vi "Filter_test.vi"(7 "Headers":string[](array[string])=["Packet Number", "Timestamp", "Source", "Destination", "Protocol", "Length", "Data"], 10 "Filter String":string="Protocol == UDP AND Length > 0.7 OR Source == 192.168.1.1", 11 "Prefiltered Data":string[][](array[string])=array1500x7[10500 elements]) -> (0 "Error Out":errorcluster, 3 "Filtered Array":string[][](array[string]))   [LabVIEW 2025, in "Table_Filtering.lvlib"]
uses:
  Table_Filtering.lvlib
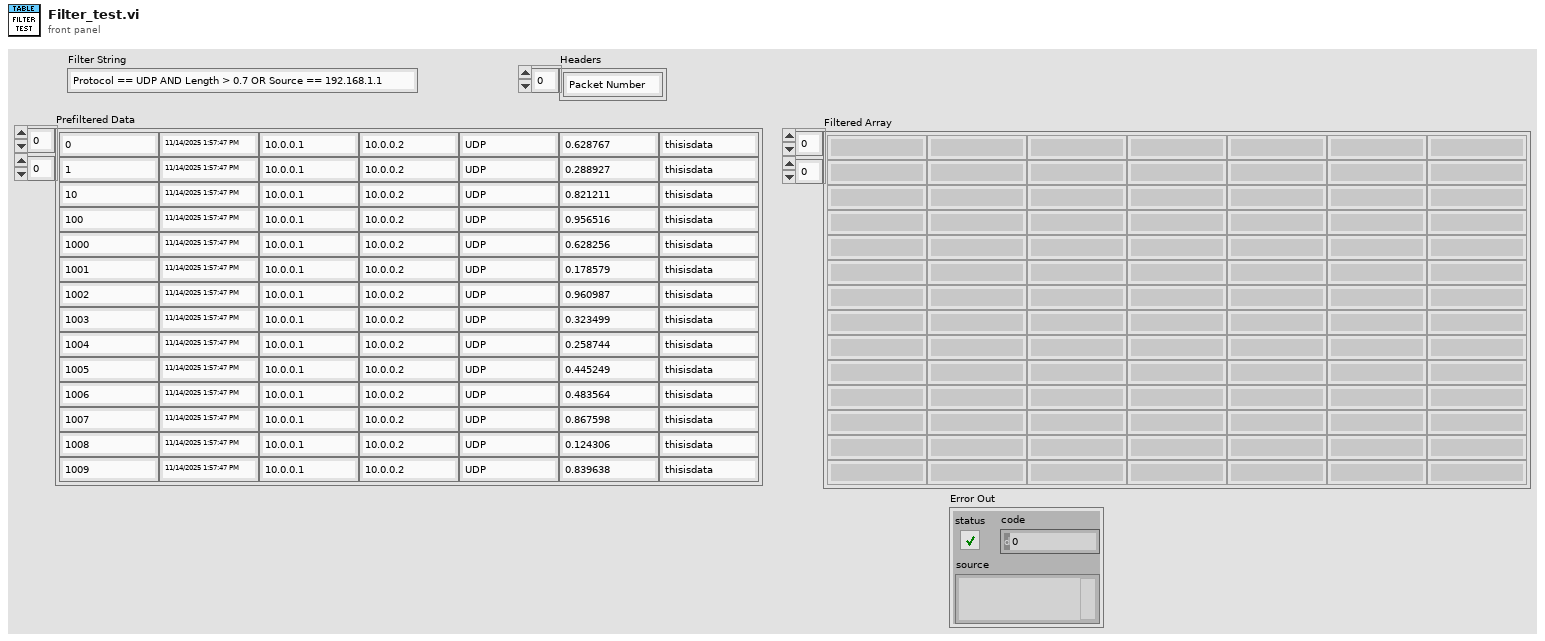
[diagram p1: front panel]
types:
  T1 = cluster{"FIELD":string, "OPERATOR":string, "VALUE":string}[]
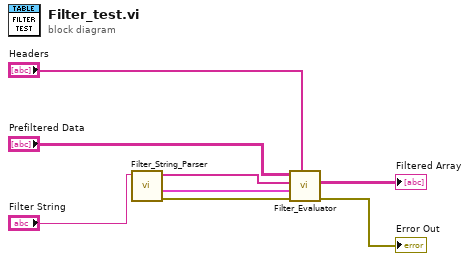
[diagram p0: block diagram]
diagram:
  n1 = call "Filter_String_Parser.vi"("Filter String"="Filter String") -> ("error constant"=w3:errorcluster, "Comparators"=w7:T1, "Boolean Connectors"=w6:string[])  [unwired: 8 in]
  n2 = call "Filter_Evaluator.vi"("Headers"="Headers", "Error"=w3, "Comparators"=w7, "Boolean Connectors"=w6, "Prefiltered Data"="Prefiltered Data") -> ("Error Out"=→"Error Out":errorcluster, "Filtered Array"=→"Filtered Array":string[][])  [unwired: 4 in, 1 out]
